vi "Get Data.vi"(8 "error in":errorcluster, 11 "TC01 in":refnum<class "TC01.lvclass">) -> (0 "error out":errorcluster, 2 "Data":dbl[](array[numeric]), 3 "TC01 out":refnum<class "TC01.lvclass">)   [LabVIEW 2015, in "TC01.lvclass"]
uses:
  TC01.lvclass
  TC01.lvclass/TC01.ctl
  <vilib>/DAQmx/read.llb/DAQmx Read (Analog DBL 1Chan 1Samp).vi
  <vilib>/DAQmx/miscellaneous.llb/DAQmx Fill In Error Info.vi
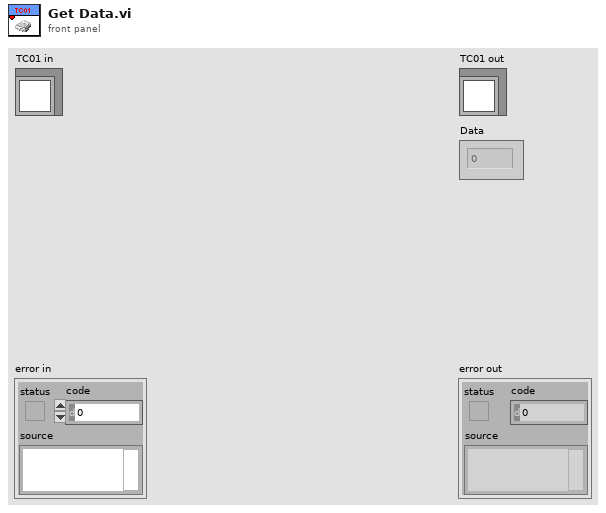
[diagram p1: front panel]
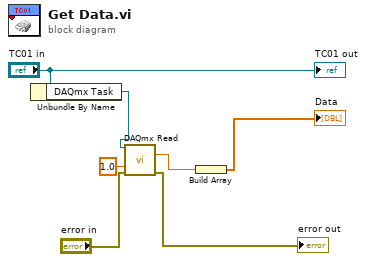
[diagram p0: block diagram]
diagram:
  n1 = Unbundle By Name("TC01 in") -> ("DAQmx Task"=w4:refnum<k21>)
  n2 = call-poly <vilib>:"DAQmx Read.vi"("task/channels in"=w4, "timeout"=1.0, "error in"="error in") -> ("data"=w6:dbl, "error out"=→"error out":errorcluster)  [unwired: 10 in, 1 out]
  n3 = Build Array(w6) -> (→"Data":dbl[])
  "TC01 out" <- "TC01 in"
